vi "STA - Wave V3 Host.vi"() -> ()   [LabVIEW 2015]
doc: "The continuous acquisition mode tells the FPGA to acquire points indefinitely until a stop command is issued or until an error is encountered (FIFO overflow, module underflow, and so on). \n\nIn this acquisition mode, explicitly call the appropriate rwfm_ConfigTiming VI and set the host application's data buffer to be many times larger than the read size. The examples use a 10X size by default. If the host application's data buffer fills, then the FPGA experiences a FIFO overflow causing the acquisition to stop."
uses:
  <vilib>/LabVIEW Targets/FPGA/cRIO/shared/nicrio_ModuleControls/nicrio_cRIO-9234_ConfigModeRing.ctl
  <vilib>/FPGAPlugInAG/cRIO-9112/niLvFpga_Open_cRIO-9112.vi
  <vilib>/rvi/interface/common/dynamic/niFpgaDynamicAddResources.vi
  <vilib>/FPGAPlugInAG/Dynamic/niLvFpga_Close_Dynamic.vi
  <vilib>/rvi/interface/nirviOpenFPGA/nirviOpenFPGA.xnode
  FPGA Bitfiles/STA-WaveformV3_FPGATarget2_[FPGA]DeltaSigMa_0miEeT0hA5U.lvbitx
  FPGA/[FPGA] DeltaSig Main V3.vi
  <vilib>/rvi/interface/nirviCloseFPGA/nirviCloseFPGA.xnode
  <vilib>/NI/cRIO Wfm/cRIO Wfm.lvlib
  D/Documents/LabVIEW Data/STA - Waveform V0/FPGA Bitfiles/SARAcqMain_9074.lvbitx
  C:/Program Files (x86)/National Instruments/LabVIEW 2015/ProjectTemplates/Source/cRIOWfm/FPGA/[FPGA] SAR Acq Main.vi
panel:
  out "data rate (S/s)":u32
  out "Channel Config":T2(array[cluster]) {"Input Configuration" items=["AC Coupled", "DC Coupled", "IEPE AC Coupled"]}
  out "Samples per Read":i32
  out "file path":path
  in  "error in (no error)":errorcluster
  out "error out":errorcluster
  in  "stop":bool
  out "Waveform Graph":waveform(sgl)[](graph)
  out "Buffer Backlog":dbl caption="RT Buffer Backlog [%]" format="%#.2g"
  # "Sampling Info"
  # "Channel Info"
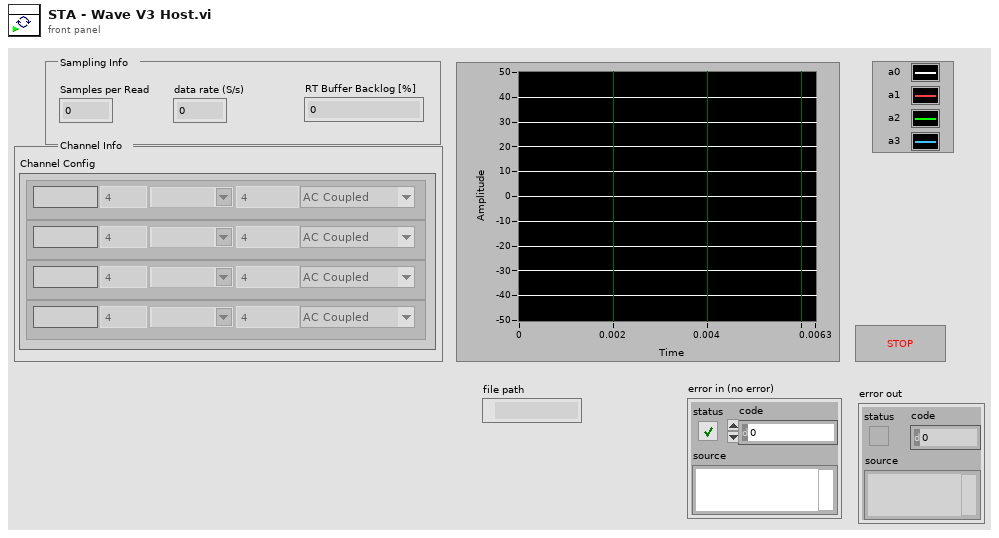
[diagram p1: front panel]
types:
  T1 = typedef "nicrio_cRIO-9234_ConfigModeRing.ctl" = u8
  T2 = cluster{"Channel Name":string, "Sensitivity mV_EU":dbl, "EU":string, "Input Configuration":T1, "dB Ref EU":dbl}[]
  T3 = enum16{"open", "open or create", "create or replace", "create", "open (read-only)"}
  T4 = typedef "Acquisition and Logging Configuration_Waveform.ctl" = cluster{"Data Rate":T5, "Samples per Read":i32, "Number of Reads to Save":i32, "Data File Name":string, "TDMS Properties":T6[], "Number of Channels":i32, "Trigger - RMS Value":dbl, "Trigger - Channel":i32, "Trigger - Time (Minute)":i32, "Channel Config":cluster{"Channel Name":string, "Sensitivity mV_EU":dbl, "EU":string, "Input Configuration":T1, "dB Ref EU":dbl}[], "data rate (S/s)":u32, "Time Measure":dbl}
  T5 = typedef "nicrio_cRIO-9234_DataRatesRing2.ctl" = u8
  T6 = typedef "TDMS Properties.ctl" = cluster{"Name":string, "Value":string}
  T7 = typedef "cRIO Wfm.lvlib/SamplingInfo.ctl" = cluster{"Number of Channels":i32, "Actual Samp Rate":dbl, "Chan Name Array":string[], "EU Chan Array":string[], "dB Ref Chan Array":dbl[]}
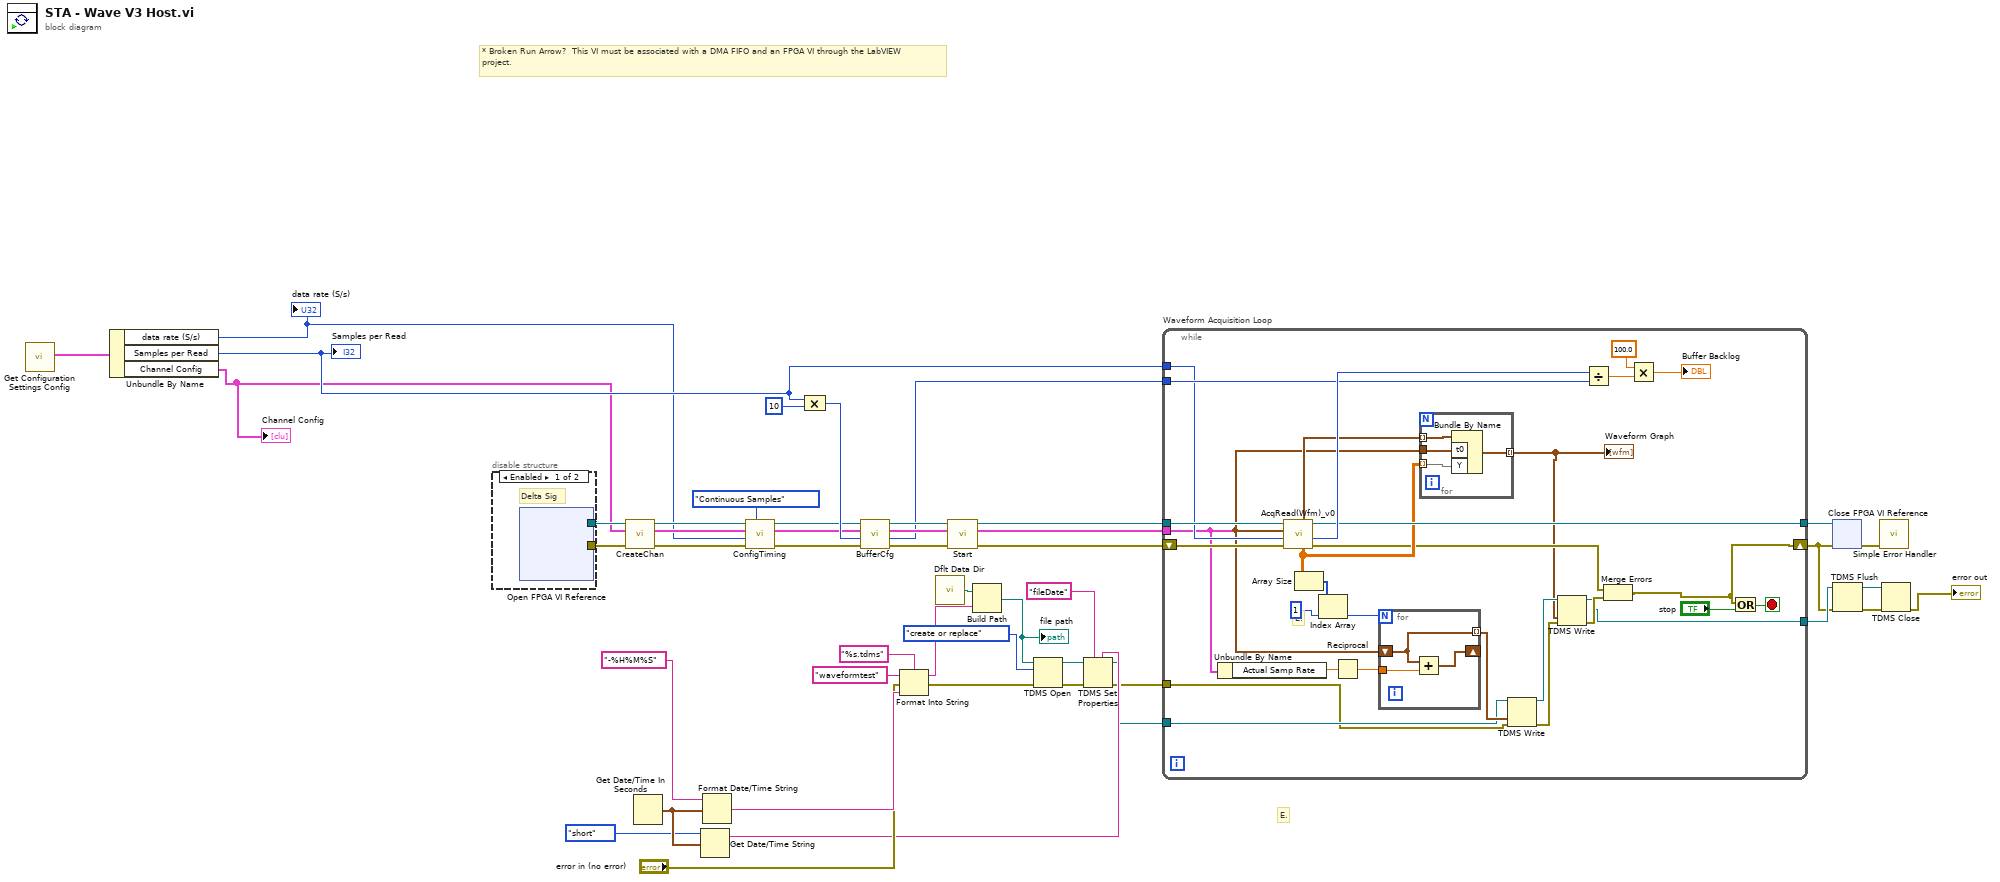
[diagram p0: block diagram]
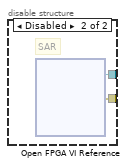
[diagram p2: hidden frame]
diagram:
  # "E."
  # "* Broken Run Arrow?  This VI must be associated with a DMA FIFO and an FPGA VI through the LabVIEW project."
  n1 = call "Get Configuration Settings Config.vi"() -> ("Configuration"=w4:T4)  [unwired: 10 in, 1 out]
  n2 = Unbundle By Name(w4) -> ("data rate (S/s)"=w1:u32, "Samples per Read"=w3:i32, "Channel Config"=w2:T2)
  "Samples per Read" <- w3
  "Channel Config" <- w2
  "data rate (S/s)" <- w1
  n3 = disable-structure shown="Enabled" {
    disable-tunnel: [w49 w51] -> w29
    disable-tunnel: [w48 w50] -> w28
    frame Enabled {
      # "Delta Sig"
      n4 = xnode "Open FPGA VI Reference"() -> ("FPGA VI Reference Out"=w49:refnum<k20>, "error out"=w48:errorcluster)  [unwired: 2 in]
    }
    frame Disabled {
      # "SAR"
      n5 = xnode "Open FPGA VI Reference"() -> ("FPGA VI Reference Out"=w51:refnum<k20>, "error out"=w50:errorcluster)  [unwired: 2 in]
    }
  }
  n6 = call <vilib>:"CreateChan.vi"("Dynamic FPGA Ref"=w29, "Channel Config"=w2, "error in"=w28) -> ("Dynamic FPGA Ref Out"=w36:refnum<k20>, "Sampling Info"=w35:T7, "error out"=w31:errorcluster)  [unwired: 5 in]
  n7 = Get Date/Time In Seconds() -> (seconds since 1Jan1904=w21:timestamp)
  n8 = Get Date/Time String(date format (0)=enum16{"short", "long", "abbreviated"}."short", seconds (now)=w21) -> (date string=w12:string)  [unwired: 1 in, 1 out]
  n9 = Format Date/Time String(time format string (%c)="-%H%M%S", seconds (now)=w21) -> (date/time string=w23:string)  [unwired: 1 in]
  n10 = call <vilib>:"ConfigTiming.vi"("Sample Mode"=enum16{"Finite Samples", "Continuous Samples"}."Continuous Samples", "error in"=w31, "Sample Rate"=w1, "Sampling Info In"=w35, "Dynamic FPGA Ref"=w36) -> ("error out"=w32:errorcluster, "Sampling Info Out"=w33:T7, "Dynamic FPGA Ref Out"=w34:refnum<k20>)  [unwired: 3 in, 1 out]
  n11 = Compound Arithmetic op=MULTIPLY(w3, 10 ("value")) -> (w40:i32)
  n12 = call <vilib>:"BufferCfg.vi"("error in"=w32, "Buffer Size [Samps per Chan]"=w40, "Sampling Info In"=w33, "Dynamic FPGA Ref"=w34) -> ("error out"=w41:errorcluster, "Buffer Size [Total Samples]"=w37:u32, "Sampling Info Out"=w39:T7, "Dynamic FPGA Ref Out"=w42:refnum<k20>)  [unwired: 4 out]
  n13 = Format Into String(format string="%s.tdms", initial string="waveformtest", error in="error in (no error)", w23) -> (resulting string=w27:string, error out=w10:errorcluster)
  n14 = call <vilib>:"Dflt Data Dir.vi"() -> ("App:Default Data Directory"=w19:path)
  n15 = call <vilib>:"Start.vi"("error in"=w41, "Sampling Info In"=w39, "Dynamic FPGA Ref"=w42) -> ("error out"=w46:errorcluster, "Sampling Info Out"=w38:T7, "Dynamic FPGA Ref Out"=w47:refnum<k20>)  [unwired: 6 out]
  n16 = Build Path(base path=w19, name or relative path=w27) -> (appended path=w15:path)
  "file path" <- w15
  n17 = TDMS Open(8:w10, 10:T3."create or replace" ("operation (0:open)"), 11:w15) -> (0:w18:errorcluster, 3:w17:refnum<k34>)  [unwired: 4 in]
  n18 = TDMS Set Properties(5:w12, 7:"fileDate" ("property names"), 8:w18, 11:w17) -> (0:w8:errorcluster, 3:w9:refnum<k34>)  [unwired: 2 in, 2 out]
  n19 = while "Waveform Acquisition Loop" {
    tunnel: w47 -> [w75]
    tunnel: [w71] -> w45
    tunnel: w38 -> [w67]
    tunnel: w37 -> [w79]
    tunnel: w3 -> [w72]
    shift-right: [w63] -> w6
    shift-left: w46 -> [w81]
    tunnel: w9 -> [w61]
    tunnel: w8 -> [w60]
    tunnel: [w56] -> w7
    stop <- w74 stop-if-true
    # "E."
    n20 = Unbundle By Name(w67) -> ("Actual Samp Rate"=w66:dbl)
    n21 = call <vilib>:"AcqRead(Wfm)_v0.vi"("error in"=w81, "Samps Read per Chan"=w72, "Sampling Info"=w67, "Dynamic FPGA Ref"=w75) -> ("error out"=w64:errorcluster, "Samples Remaining"=w80:u32, "time stamp"=w68:timestamp, "Dynamic FPGA Ref Out"=w71:refnum<k20>, "transposed array"=w69:sgl[][], "Array"=w70:waveform(sgl)[])  [unwired: 2 in]
    n22 = Array Size(array=w69) -> (size(s)=w55:i32[])
    n23 = Index Array(array=w55, index=1) -> (element=w53:i32)
    n24 = Reciprocal(x=w66) -> (1/x=w65:dbl)
    n25 = for {
      N: w53 -> [_]
      shift-right: [w84] -> _
      shift-left: w68 -> [w83]
      tunnel: [w83] -> w62 mode=indexing
      tunnel: w65 -> [w82]
      n26 = Add(x=w83, y=w82) -> (x+y=w84:timestamp)
    }
    n27 = for {
      tunnel: w70 -> [w88] mode=indexing
      tunnel: w68 -> [w87]
      tunnel: [w86] -> w52 mode=indexing
      tunnel: w69 -> [w85] mode=indexing
      n28 = Bundle By Name(cluster=w88, "t0"=w87, "Y"=w85) -> (w86:waveform(sgl))
    }
    "Waveform Graph" <- w52
    n29 = TDMS Write(0:w61, 9:w62, 11:w60) -> (4:w58:refnum<k34>, 15:w59:errorcluster)  [unwired: 3 in, 2 out]
    n30 = TDMS Write(0:w58, 9:w52, 11:w59) -> (4:w56:refnum<k34>, 15:w57:errorcluster)  [unwired: 3 in, 2 out]
    n31 = Divide(x=w80, y=w79) -> (x/y=w78:dbl)
    n32 = Merge Errors(w64, w57) -> (w63:errorcluster)
    n33 = Multiply(x=100.0, y=w78) -> (x*y=→"Buffer Backlog":dbl)
    n34 = Or(x=w63, y="stop") -> (x .or. y?=w74:bool)
  }
  n35 = xnode "Close FPGA VI Reference"("FPGA VI Reference In"=w45, "error in"=w6) -> ("error out"=w43:errorcluster)
  n36 = TDMS Flush(4:w6, 7:w7) -> (0:w16:errorcluster, 3:w5:refnum<k34>)
  n37 = call <vilib>:"Simple Error Handler.vi"("error in (no error)"=w43) -> ()  [unwired: 1 in, 8 out]
  n38 = TDMS Close(8:w16, 11:w5) -> (0:→"error out":errorcluster)  [unwired: 1 out]
